vi "OnOffGenParametr (SubVI).vi"(4 "DigNum Refnum 3":refnum<vi>, 5 "OnnOffGen":bool, 6 "Bool Refnum 2":refnum<vi>, 7 "DigNum Refnum":refnum<vi>, 9 "Bool Refnum":refnum<vi>, 10 "DigNum Refnum 2":refnum<vi>, 11 "Digital in":refnum<vi>) -> ()   [LabVIEW 2017]
uses:
  st_str Global.vi
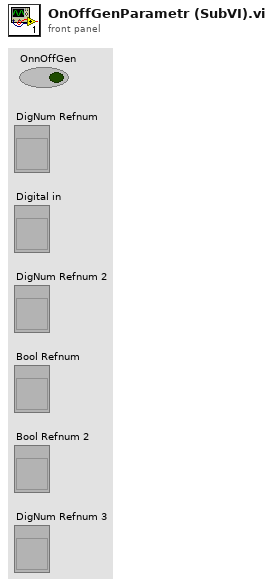
[diagram p1: front panel]
types:
  T1 = enum8{"Enabled", "Disabled", "Disabled and Grayed Out"}
  T2 = typedef "A5000_param.ctl" = cluster{"ChannelA":cluster{"Enabled":bool, "Coupling":i16, "Range":u16, "Analogue Offset":sgl}, "ChannelB":cluster{"Enabled":bool, "Coupling":i16, "Range":u16, "Analogue Offset":sgl}, "Trigger":cluster{"Trigger Enabled":bool, "Trigger Source":enum16{"Channel A", "Channel B", "Channel C", "Channel D", "Ext."}, "Trigger Threshold (volts)":dbl, "Trigger Direction":u16, "Trigger Delay (samples)":u32, "Auto Trigger Time (ms)":i16}, "MaxADCvalue":i16, "handle":i16, "Acquisition":cluster{"preTriggerSamples":i32, "postTriggerSamples":i32, "timebase":u32, "Down-Sample Mode":u32, "Down Sample Ratio":u32}, "Device Info":cluster{"Driver Version":string, "USB Version":string, "Hardware":string, "Variant":string, "Batch and Serial":string, "Cal Date":string, "Kernel Version":string, "Digital HW Version":string, "Analogue HW Version":string, "MSO":bool, "Number of channels":i16}, "Properties":cluster{"Sample Frequency":sgl, "Sample Rate":sgl, "Max Samples Available":i32, "Number of Samples":u32, "Total Capture Time (sec) ":sgl, "Max Total Capture Time Available (sec)":sgl}, "Resolution":i32, "EmulateV":bool, "General AWG Settings":cluster{"Peak-to-Peak Voltage (microvolts)":u32, "Offset Voltage (microvolts)":i32, "Wave Type":u32, "Sweep Type":u32, "Shots":u32, "Sweeps":u32, "Trigger Type":u32, "Trigger Source":u32, "Ext. Threshold (ADC count)":i16, "White Noise/PRBS":u32}, "Standard Waveform Settings":cluster{"Start Frequency":dbl, "Stop Frequency":dbl, "Increment":dbl, "Dwell Time (seconds)":dbl}, "Arbitrary Waveform Settings":cluster{"Arbirary waveform file path":path, "Index Mode":u32}, "AutoDiapChA":bool, "AutoDiapChB":bool}
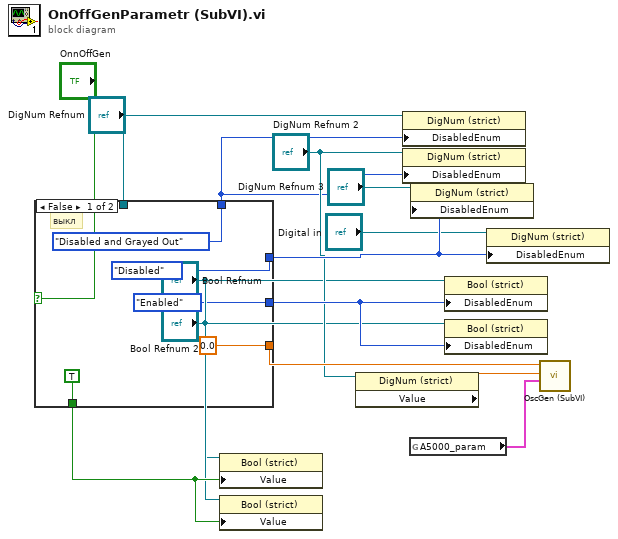
[diagram p0: block diagram]
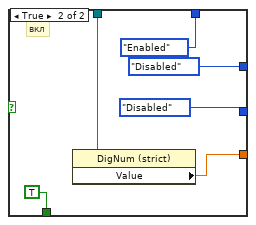
[diagram p2: hidden frame]
diagram:
  n1 = case shown="False" "OnnOffGen" {
    tunnel: [0.0 ("VChGEN") w25] -> w10
    tunnel: [TRUE TRUE] -> w11
    tunnel: [T1."Disabled and Grayed Out" ("Disabled") T1."Enabled" ("Disabled")] -> w1
    tunnel: [T1."Disabled" ("Disabled") T1."Disabled" ("Disabled")] -> w12
    tunnel: [T1."Enabled" ("Disabled") T1."Disabled" ("Disabled")] -> w13
    tunnel: "DigNum Refnum" -> [_ w20]
    frame False {
      # "выкл"
    }
    frame True {
      # "вкл"
      n2 = property class="DigNum (strict)"(reference=w20) -> ("Value"=w25:dbl)  [unwired: 1 in, 2 out]
    }
  }
  n3 = property on="Property Node" class="Bool (strict)"(reference="Bool Refnum 2", "Value"=w11) -> ()  [unwired: 1 in, 2 out]
  n4 = property on="Property Node" class="Bool (strict)"(reference="Bool Refnum", "Value"=w11) -> ()  [unwired: 1 in, 2 out]
  n5 = property class="DigNum (strict)"(reference="DigNum Refnum 2") -> ("Value"=w9:dbl)  [unwired: 1 in, 2 out]
  n6 = property on="Property Node" class="DigNum (strict)"(reference="DigNum Refnum", "DisabledEnum"=w1) -> ()  [unwired: 1 in, 2 out]
  n7 = property on="Property Node" class="DigNum (strict)"(reference="DigNum Refnum 2", "DisabledEnum"=w1) -> ()  [unwired: 1 in, 2 out]
  n8 = global read "st_str Global.vi" "A5000_param"() -> (w8:T2)
  n9 = property on="Property Node" class="DigNum (strict)"(reference="DigNum Refnum 3", "DisabledEnum"=w12) -> ()  [unwired: 1 in, 2 out]
  n10 = property on="Property Node" class="Bool (strict)"(reference="Bool Refnum", "DisabledEnum"=w13) -> ()  [unwired: 1 in, 2 out]
  n11 = property on="Property Node" class="Bool (strict)"(reference="Bool Refnum 2", "DisabledEnum"=w13) -> ()  [unwired: 1 in, 2 out]
  n12 = property on="Property Node" class="DigNum (strict)"(reference="Digital in", "DisabledEnum"=w12) -> ()  [unwired: 1 in, 2 out]
  n13 = call "OscGen (SubVI).vi"("A5000_param_out"=w8, "Frequency,kHz"=w9, "UgenVrms"=w10) -> ()  [unwired: 8 in, 1 out]
